vi "Creat AOs.vi"(0 "reference in":refnum<class "Stand.lvclass">, 11 "error in (no error)":errorcluster) -> (4 "reference out":refnum<class "Stand.lvclass">, 15 "error out":errorcluster)   [LabVIEW 2019, in "Stand.lvclass"]
uses:
  Stand.lvclass
  C:/Users/ANENKOV_V1/Desktop/src/Proccess_class/Proccess.lvclass
  Stand.lvclass/Stand.ctl
  Proccess_class/Proccess.lvclass/Proccess.ctl
  Proccess_class/TAGs.ctl
  AO_class/AO.lvclass
  Proccess_class/Proccess.lvclass
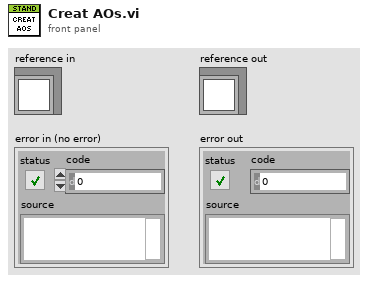
[diagram p1: front panel]
types:
  T1 = typedef "Proccess.lvclass/TAGs.ctl" = cluster{"TAG":string, "PTAG":string, "DESC":string}
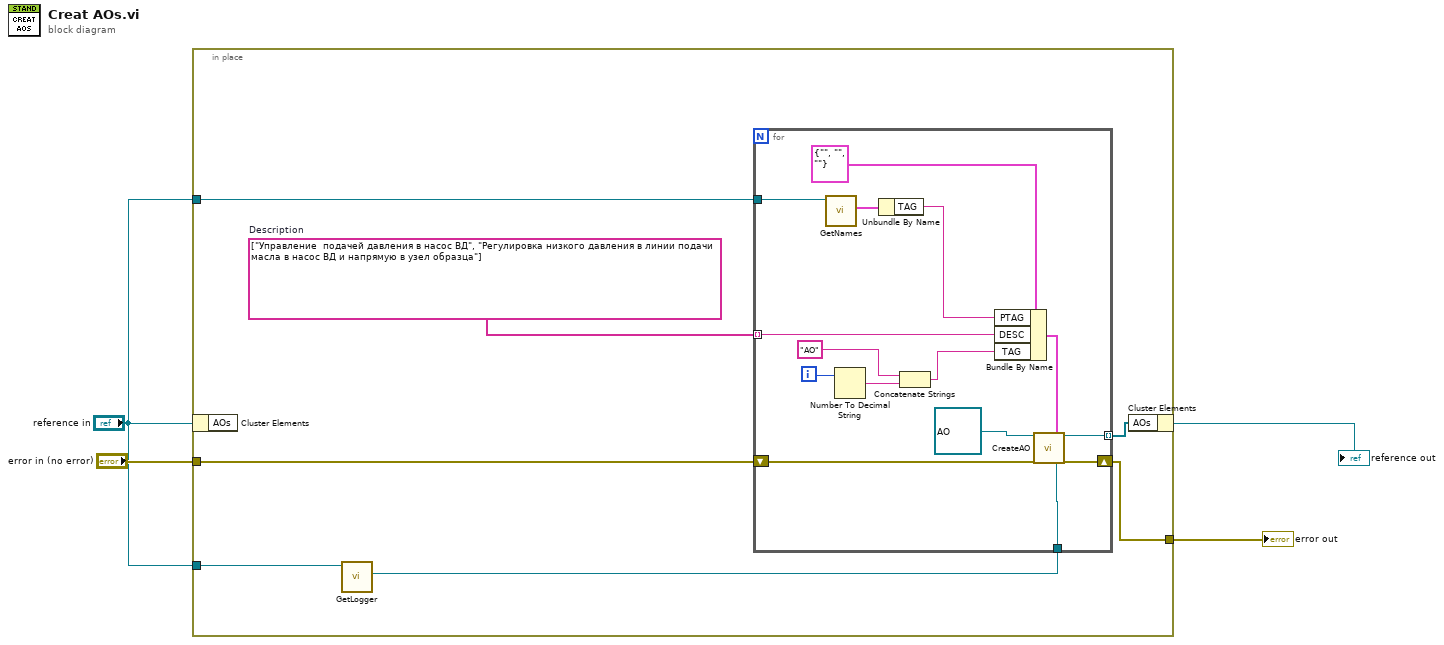
[diagram p0: block diagram]
diagram:
  n1 = in-place {
    in-place-border: "error in (no error)" -> [w11]
    in-place-border: "reference in" -> [w9]
    in-place-border: "reference in" -> [w8]
    in-place-border: [w5] -> w4
    w6 = string[] ["Управление  подачей давления в насос ВД", "Регулировка низкого давления в линии подачи масла в насос ВД и напрямую в узел образца"]  # Description
    n2 = in-place-cluster #1("reference in") -> ()  [unwired: 1 out]
    n3 = call "GetLogger.vi"("Proccess in"=w8) -> ("Logger"=w7:refnum<class "Logger.lvclass">)  [unwired: 10 in]
    n4 = for {
      tunnel: [w13] -> w10 mode=indexing
      shift-right: [w12] -> w5
      shift-left: w11 -> [w15]
      tunnel: w6 -> [w21] mode=indexing
      tunnel: w9 -> [w18]
      tunnel: w7 -> [w14]
      i -> [w26]
      n5 = call "GetNames.vi"("Proccess in"=w18) -> ("Tags"=w20:T1)  [unwired: 10 in]
      n6 = Number To Decimal String(number=w26) -> (decimal integer string=w25:string)  [unwired: 1 in]
      n7 = Unbundle By Name(w20) -> ("TAG"=w19:string)
      n8 = Concatenate Strings("AO" ("string"), w25) -> (w22:string)
      n9 = Bundle By Name(cluster=T1 {"TAG"="", "PTAG"="", "DESC"=""} ("Tags"), "PTAG"=w19, "DESC"=w21, "TAG"=w22) -> (w17:T1)
      n10 = call "CreateAO.vi"("AI in"=refnum<class "AO.lvclass"> refnum, "error in (no error)"=w15, "Tags"=w17, "Logger"=w14) -> ("AI out"=w13:refnum<class "AO.lvclass">, "error out"=w12:errorcluster)  [unwired: 14 in]
    }
    n11 = in-place-cluster #1("AOs"=w10) -> (→"reference out":refnum<class "Stand.lvclass">)
  }
  "error out" <- w4
